vi "GetBacklogForListenerProcess.vi"(8 "error in (no error)":errorcluster, 10 "process name":string, 11 "Qbus in":refnum<class "Qbus.lvclass">) -> (0 "error in (no error)":errorcluster, 1 "# elements in queue":i32, 3 "Qbus out":refnum<class "Qbus.lvclass">)   [LabVIEW 2017, in "Qbus.lvclass"]
uses:
  <vilib>/addons/Qbus/Qbus.lvclass
  <vilib>/addons/Qbus/Qbus.lvclass/Qbus.ctl
  <vilib>/addons/Qbus/controls/message.ctl
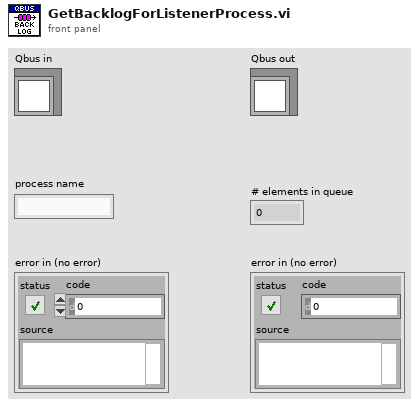
[diagram p1: front panel]
types:
  T1 = typedef "Qbus.lvclass/data.ctl" = cluster{"Queues":variant, "Subscriptions":variant, "MasterQ":string}
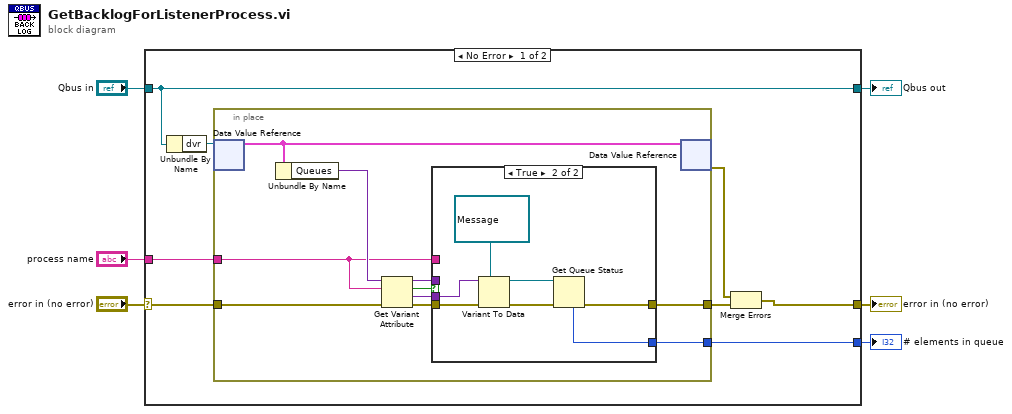
[diagram p0: block diagram]
diagram:
  n1 = case shown="No Error" "error in (no error)" {
    selector: "error in (no error)" -> [w10 w34]
    tunnel: [w9 w34] -> w5
    tunnel: [w14 w33] -> w3
    tunnel: "Qbus in" -> [w14 w33]
    tunnel: "process name" -> [w12 _]
    tunnel: [w7 _] -> w1
    frame No Error {
      n2 = Unbundle By Name(w14) -> ("dvr"=w13:refnum<data-value>)
      n3 = in-place {
        in-place-border: w10 -> [w24]
        in-place-border: w12 -> [w19]
        in-place-border: [w18] -> w8
        in-place-border: [w15] -> w7
        n4 = in-place-dvr #1(w13) -> (w17:T1)  [unwired: 1 out]
        n5 = Unbundle By Name(w17) -> ("Queues"=w21:variant)
        n6 = Get Variant Attribute(Variant=w21, name=w19, error in=w24) -> (duplicate Variant=w20:variant, found=w23:bool, value=w16:variant, error out=w22:errorcluster)  [unwired: 1 in]
        n7 = case shown="True" w23 {
          tunnel: w22 -> [w25 w32]
          tunnel: w20 -> [_ _]
          tunnel: w19 -> [_ _]
          tunnel: [w25 w27] -> w18
          tunnel: w16 -> [_ w31]
          tunnel: [_ w26] -> w15
          frame False {
          }
          frame True {
            n8 = Variant To Data(error in=w32, type=refnum<queue> refnum ("queue out"), Variant=w31) -> (data=w29:refnum<queue>, error out=w28:errorcluster)
            n9 = Get Queue Status(queue=w29, error in (no error)=w28) -> (error out=w27:errorcluster, # elements in queue=w26:i32)  [unwired: 1 in, 6 out]
          }
        }
        n10 = in-place-dvr #1(w17) -> (w11:errorcluster)  [unwired: 1 out]
      }
      n11 = Merge Errors(w11, w8) -> (w9:errorcluster)
    }
    frame Error {
    }
  }
  "error in (no error)" <- w5
  "Qbus out" <- w3
  "# elements in queue" <- w1
